vi "task2.3.vi"() -> ()   [LabVIEW 2021]
doc: "This example demonstrates how to continuously re-generate analog output data from a buffer in your computer's memory.\n\nRefer to your device documentation for pinouts and hardware capabilities."
uses:
  <vilib>/DAQmx/write.llb/DAQmx Write (Analog Wfm 1Chan NSamp).vi
  <vilib>/DAQmx/write.llb/DAQmx Write (Digital Bool 1Line 1Point).vi
  <vilib>/DAQmx/read.llb/DAQmx Read (Analog 1D Wfm NChan NSamp).vi
  <vilib>/DAQmx/create/channels.llb/DAQmx Create Channel (AO-Voltage-Basic).vi
  <vilib>/DAQmx/configure/timing.llb/DAQmx Timing (Sample Clock).vi
  <vilib>/DAQmx/create/channels.llb/DAQmx Create Channel (AI-Voltage-Basic).vi
  <vilib>/DAQmx/configure/trigger.llb/DAQmx Start Trigger (Digital Edge).vi
  <vilib>/DAQmx/miscellaneous.llb/DAQmx Fill In Error Info.vi
  <vilib>/DAQmx/create/channels.llb/DAQmx Create Channel (DO-Digital Output).vi
  <vilib>/measure/matone.llb/Extract Single Tone Information N Chan.vi
  <vilib>/Waveform/WDTFileIO.llb/ Write Waveform to File.vi
  <vilib>/Waveform/WDTFileIO.llb/ Write Waveforms to File (1D).vi
  <vilib>/express/express analysis/Spectral/Block/exnSpectralBlock spectral measurements peak poly.vi
  <vilib>/express/express analysis/Spectral/Block/exnSpectralBlock spectral measurements peak array WFM.vi
  <vilib>/express/express analysis/Spectral/Block/exnSpectralBlock spectral measurements peak WFM.vi
  <vilib>/express/express analysis/Spectral/XNode/ExpressSpectralMeasurementsBlockNode.xnode
  <vilib>/measure/NI_MABase.lvlib
  <vilib>/measure/NI_MAPro.lvlib
panel:
  out "A1 frequency (db) 2":dbl=0.03331269437933233
  out "A1 amplitude (db)":dbl=0.03331269437933233
  out "A1 phase (deg)":dbl=264.9568956886852
  out "Output Freq":cluster{"f0":dbl, "df":dbl, "magnitude":dbl[]}(graph)
  out "Input Freq":cluster{"f0":dbl, "df":dbl, "magnitude":dbl[]}[](graph)
  in  "Amplitude":dbl=1.0 format="%0.2p"
  in  "Frequency":dbl=10.0 format="%0.2p"
  in  "Waveform Type":u16(ring) items=["Sine Wave", "Triangle Wave", "Square Wave", "Sawtooth Wave"]
  in  "Input Channel 2":tag="Dev3/ai1"
  in  "Number of samples":i32=1000
  out "Input Voltage":waveform(dbl)[](graph)=[{"t0"=timestamp(3702416907.610318 s since 1904-01-01), "dt"=9.999999999999999e-05, "Y"=array[1000 elements], "attributes"=variant("NI_ChannelName"=variant(string "Dev6/ai0"), "NI_UnitDescription"=variant(string "Volts"))}, {"t0"=timestamp(3702416907.610332 s since 1904-01-01), "dt"=9.999999999999999e-05, "Y"=array[1000 elements], "attributes"=variant("NI_ChannelName"=variant(string "Dev6/ai1"), "NI_UnitDescription"=variant(string "Volts"))}]
  in  "Input Channel 1":tag="Dev3/ai0"
  in  "Min Input Voltage":dbl=-10.0
  in  "Max Input Voltage":dbl=10.0
  in  "Output sample rate":dbl=10000.0 format="%0.2f"
  out "Output Voltage":waveform(dbl)(graph)={"t0"=timestamp(0 s since 1904-01-01), "dt"=0.0001, "Y"=array[1000 elements]}
  in  "Max Voltage":dbl=10.0
  in  "Min Voltage":dbl=-10.0
  in  "Output Channel":tag="Dev3/ao0"
  # "Output Channel Settings"
  # "Output voltage"
  # "Input voltage"
  # "Input Channel Settings"
  # "Waveform Settings"
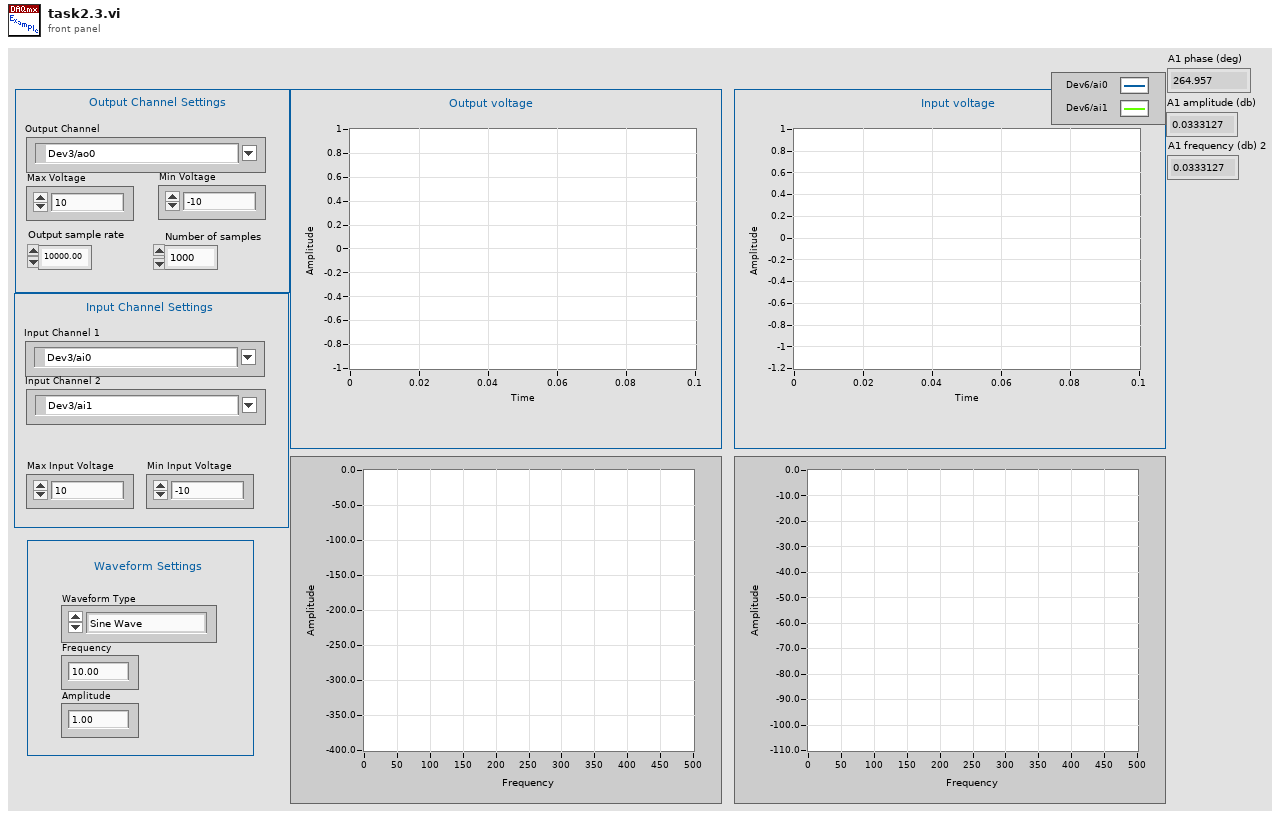
[diagram p1: front panel]
types:
  T1 = cluster{"Output sample rate":dbl, "Number of samples":i32}
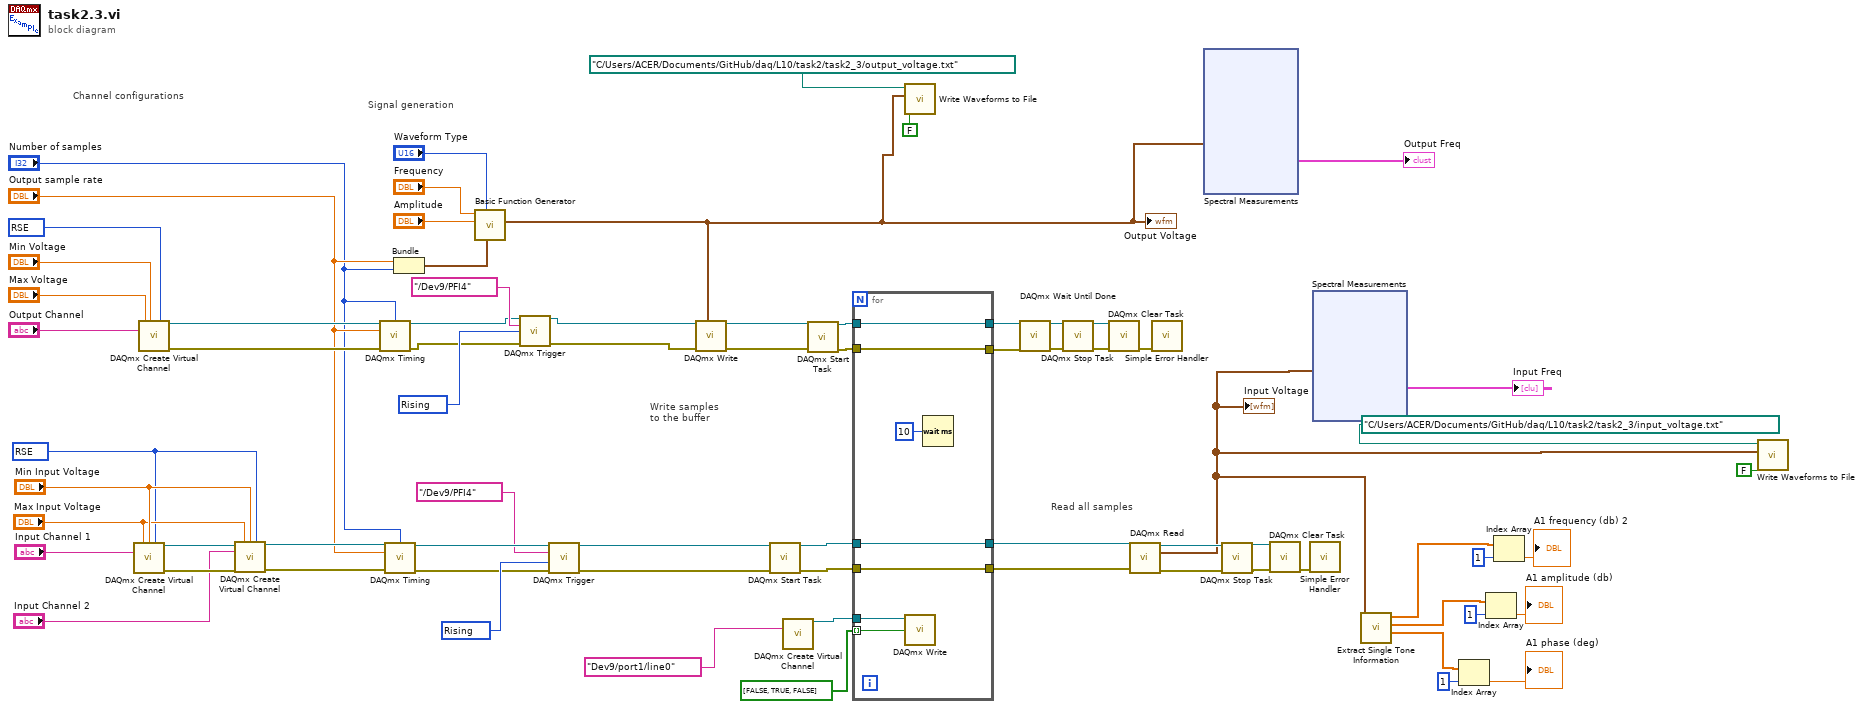
[diagram p0: block diagram]
diagram:
  w20 = 10280 items=["Rising"=10280, "Falling"=10171] ("edge")
  w24 = 10280 items=["Rising"=10280, "Falling"=10171] ("edge")
  w48 = 10083 items=["Default"=-1, "RSE"=10083, "NRSE"=10078, "Differential"=10106, "Pseudodifferential"=12529] ("input terminal configuration")
  w62 = 10083 items=["Default"=-1, "RSE"=10083, "NRSE"=10078, "Differential"=10106, "Pseudodifferential"=12529] ("input terminal configuration")
  # "Read all samples"
  # "Write samples\nto the buffer"
  # "Signal generation"
  # "Channel configurations"
  n1 = call-poly <vilib>:"DAQmx Create Virtual Channel.vi"("maximum value"="Max Input Voltage", "minimum value"="Min Input Voltage", "input terminal configuration"=w48, "physical channels"="Input Channel 1") -> ("task out"=w58:refnum<k21>, "error out"=w59:errorcluster)  [unwired: 10 in]
  n2 = call-poly <vilib>:"DAQmx Create Virtual Channel.vi"("maximum value"="Max Voltage", "minimum value"="Min Voltage", "output terminal configuration"=w62, "physical channels"="Output Channel") -> ("task out"=w66:refnum<k21>, "error out"=w67:errorcluster)  [unwired: 10 in]
  n3 = call-poly <vilib>:"DAQmx Create Virtual Channel.vi"("task in"=w58, "maximum value"="Max Input Voltage", "minimum value"="Min Input Voltage", "input terminal configuration"=w48, "physical channels"="Input Channel 2", "error in"=w59) -> ("task out"=w57:refnum<k21>, "error out"=w56:errorcluster)  [unwired: 8 in]
  n4 = call-poly <vilib>:"DAQmx Timing.vi"("task/channels in"=w66, "samples per channel"="Number of samples", "rate"="Output sample rate", "error in"=w67) -> ("task out"=w25:refnum<k21>, "error out"=w23:errorcluster)  [unwired: 10 in]
  n5 = call-poly <vilib>:"DAQmx Timing.vi"("task/channels in"=w57, "samples per channel"="Number of samples", "rate"="Output sample rate", "error in"=w56) -> ("task out"=w17:refnum<k21>, "error out"=w19:errorcluster)  [unwired: 10 in]
  n6 = Bundle "Bundle"("Output sample rate"="Output sample rate", "Number of samples"="Number of samples") -> (w47:T1)  [unwired: 1 in]
  n7 = call <vilib>:"Basic Function Generator.vi"("sampling info"=w47, "signal type"="Waveform Type", "amplitude"="Amplitude", "frequency"="Frequency") -> ("signal out"=w11:waveform(dbl))  [unwired: 5 in, 2 out]
  "Output Voltage" <- w11
  n8 = call-poly <vilib>:"DAQmx Trigger.vi"("task/channels in"=w25, "source"=tag "/Dev9/PFI4", "edge"=w24, "error in"=w23) -> ("task out"=w28:refnum<k21>, "error out"=w27:errorcluster)  [unwired: 10 in]
  n9 = call-poly <vilib>:"DAQmx Trigger.vi"("task/channels in"=w17, "source"=tag "/Dev9/PFI4", "edge"=w20, "error in"=w19) -> ("task out"=w22:refnum<k21>, "error out"=w21:errorcluster)  [unwired: 10 in]
  n10 = call-poly <vilib>:"DAQmx Write.vi"("task/channels in"=w28, "data"=w11, "error in"=w27) -> ("task out"=w30:refnum<k21>, "error out"=w29:errorcluster)  [unwired: 10 in, 1 out]
  n11 = call <vilib>:"DAQmx Start Task.vi"("task/channels in"=w22, "error in"=w21) -> ("task out"=w37:refnum<k21>, "error out"=w38:errorcluster)  [unwired: 12 in]
  n12 = call-poly <vilib>:"DAQmx Create Virtual Channel.vi"("lines"=tag "Dev9/port1/line0") -> ("task out"=w35:refnum<k21>)  [unwired: 13 in, 1 out]
  n13 = call <vilib>:"DAQmx Start Task.vi"("task/channels in"=w30, "error in"=w29) -> ("task out"=w39:refnum<k21>, "error out"=w40:errorcluster)  [unwired: 12 in]
  n14 = for {
    tunnel: bool[] [FALSE, TRUE, FALSE] -> [w79] mode=indexing
    tunnel: w38 -> [w75]
    tunnel: w37 -> [w76]
    tunnel: w40 -> [w77]
    tunnel: w39 -> [w78]
    tunnel: [w78] -> w34
    tunnel: [w77] -> w33
    tunnel: [w76] -> w32
    tunnel: [w75] -> w31
    tunnel: w35 -> [w74]
    n15 = call-poly <vilib>:"DAQmx Write.vi"("task/channels in"=w74, "data"=w79) -> ()  [unwired: 11 in, 3 out]
    n16 = Wait (ms)(milliseconds to wait=u32 10) -> ()  [unwired: 1 out]
  }
  n17 = call-poly <vilib>:"Write Waveforms to File.vi"("append to file? (new file:F)"=FALSE, "waveform"=w11, "file path (dialog if empty)"=path "C:/Users/ACER/Documents/GitHub/daq/L10/task2/task2_3/output_voltage.txt") -> ()  [unwired: 7 in, 2 out]
  n18 = call <vilib>:"DAQmx Wait Until Done.vi"("task/channels in"=w34, "error in"=w33) -> ("task out"=w44:refnum<k21>, "error out"=w43:errorcluster)  [unwired: 12 in]
  n19 = call <vilib>:"DAQmx Stop Task.vi"("task/channels in"=w44, "error in"=w43) -> ("task out"=w69:refnum<k21>, "error out"=w68:errorcluster)  [unwired: 12 in]
  n20 = call <vilib>:"DAQmx Clear Task.vi"("task in"=w69, "error in"=w68) -> ("error out"=w73:errorcluster)  [unwired: 13 in]
  n21 = call-poly <vilib>:"DAQmx Read.vi"("task/channels in"=w32, "error in"=w31) -> ("task out"=w60:refnum<k21>, "data"=w1:waveform(dbl)[], "error out"=w61:errorcluster)  [unwired: 11 in]
  "Input Voltage" <- w1
  n22 = call <vilib>:"Simple Error Handler.vi"("error in (no error)"=w73) -> ()  [unwired: 4 in, 5 out]
  n23 = xnode "Spectral Measurements"("Signals"=w11) -> ("FFT - (Peak)"=→"Output Freq":cluster{"f0":dbl, "df":dbl, "magnitude":dbl[]})  [unwired: 1 in, 2 out]
  n24 = call <vilib>:"DAQmx Stop Task.vi"("task/channels in"=w60, "error in"=w61) -> ("task out"=w64:refnum<k21>, "error out"=w65:errorcluster)  [unwired: 12 in]
  n25 = call <vilib>:"DAQmx Clear Task.vi"("task in"=w64, "error in"=w65) -> ("error out"=w63:errorcluster)  [unwired: 13 in]
  n26 = call <vilib>:"Simple Error Handler.vi"("error in (no error)"=w63) -> ()  [unwired: 4 in, 5 out]
  n27 = xnode "Spectral Measurements"("Signals"=w1) -> ("FFT - (Peak)"=→"Input Freq":cluster{"f0":dbl, "df":dbl, "magnitude":dbl[]}[])  [unwired: 1 in, 2 out]
  n28 = call-poly <vilib>:"Extract Single Tone Information.vi"("time signals in"=w1) -> ("detected phases (deg)"=w7:dbl[], "detected amplitudes"=w9:dbl[], "detected frequencies"=w2:dbl[])  [unwired: 5 in, 3 out]
  n29 = Index Array(array=w7, index=1) -> (element=→"A1 phase (deg)":dbl)
  n30 = Index Array(array=w9, index=1) -> (element=→"A1 amplitude (db)":dbl)
  n31 = Index Array(array=w2, index=1) -> (element=→"A1 frequency (db) 2":dbl)
  n32 = call-poly <vilib>:"Write Waveforms to File.vi"("append to file? (new file:F)"=FALSE, "waveform array"=w1, "file path (dialog if empty)"=path "C:/Users/ACER/Documents/GitHub/daq/L10/task2/task2_3/input_voltage.txt") -> ()  [unwired: 7 in, 2 out]
